vi "Arrow Rotate Angle.vi"(11 "Vector":cluster{"X":sgl, "Y":sgl, "Z":sgl}) -> (1 "Z Axis Rotate Angle":sgl, 2 "Y Axis Rotate Angle":sgl)   [LabVIEW 2020, in "3D Quiver.lvclass"]
uses:
  <vilib>/Math Plots/3D Math Plots/3D Quiver/3D Quiver/3D Quiver.lvclass
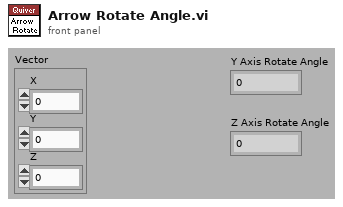
[diagram p1: front panel]
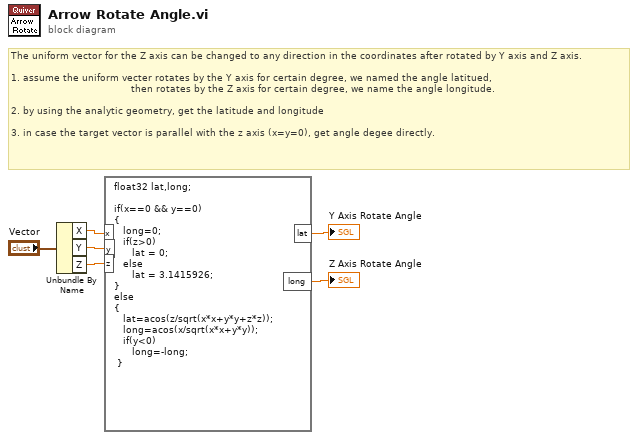
[diagram p0: block diagram]
diagram:
  # "The uniform vector for the Z axis can be changed to any direction in the coordinates after rotated by Y axis and Z axis.\n\n1. assume the uniform vecter rotates by the Y axis for certain degree, we named the angle latitued,\n                                        then rotates by the Z axis for certain degree, we name the angle longitude.\n\n2. by using the analytic geometry, get the latitude and longitude\n\n3. in case the target vector is parallel with the z axis (x=y=0), get angle degee directly."
  n1 = Unbundle By Name("Vector") -> ("X"=w3:sgl, "Y"=w2:sgl, "Z"=w1:sgl)
  n2 = formula code="float32 lat,long;\n\nif(x==0 && y==0)\n{\n   long=0;\n   if(z>0)\n      lat = 0;\n   else\n      lat = 3.1415926;\n}\nelse\n{\n   lat=acos(z/sqrt(x*x+y*y+z*z));\n   long=acos(x/sqrt(x*x+y*y));\n   if(y<0)\n      long=-long;\n }"("x"=w3, "y"=w2, "z"=w1) -> ("lat"=→"Y Axis Rotate Angle":sgl, "long"=→"Z Axis Rotate Angle":sgl)
